vi "Run.vi"(7 "Team Index":i32, 8 "Column":i32, 9 "Row":i32, 10 "View":i32[](array[numeric]) caption="View (Team Index, -1: empty)", 11 "Uno In":refnum<class "Uno.lvclass">) -> (0 "Replicated":refnum<class "Square.lvclass">, 1 "Direction":T1, 2 "Action":T2, 3 "Square Out":refnum<class "Square.lvclass">)   [LabVIEW 2017, in "Uno.lvclass"]
uses:
  Uno.lvclass
  C:/Workspace/Endigit/SquareBattle/Square/Square.lvclass
  Square/Square.lvclass
  Type Defs/Action Enum.ctl
  Type Defs/Direction Enum.ctl
  Uno.lvclass/Uno.ctl
  Finish/Finish.lvclass
  SubVIs/Read-Only Globals.vi
  SubVIs/Read-Only Stats.vi
  SubVIs/Globals (private).vi
  Type Defs/SB Type Defs.lvlib
panel:
  # "NW\nN\nNE\nE\nSE\nS\nSW\nW"
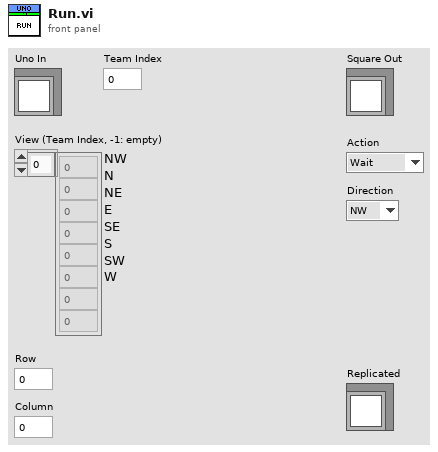
[diagram p1: front panel]
types:
  T1 = typedef "SB Type Defs.lvlib/Direction Enum.ctl" = enum16{"NW", "N", "NE", "E", "SE", "S", "SW", "W"}
  T2 = typedef "SB Type Defs.lvlib/Action Enum.ctl" = enum16{"Wait", "Move", "Attack", "Replicate"}
  T3 = typedef "Semaphore RefNum" = refnum<k1>
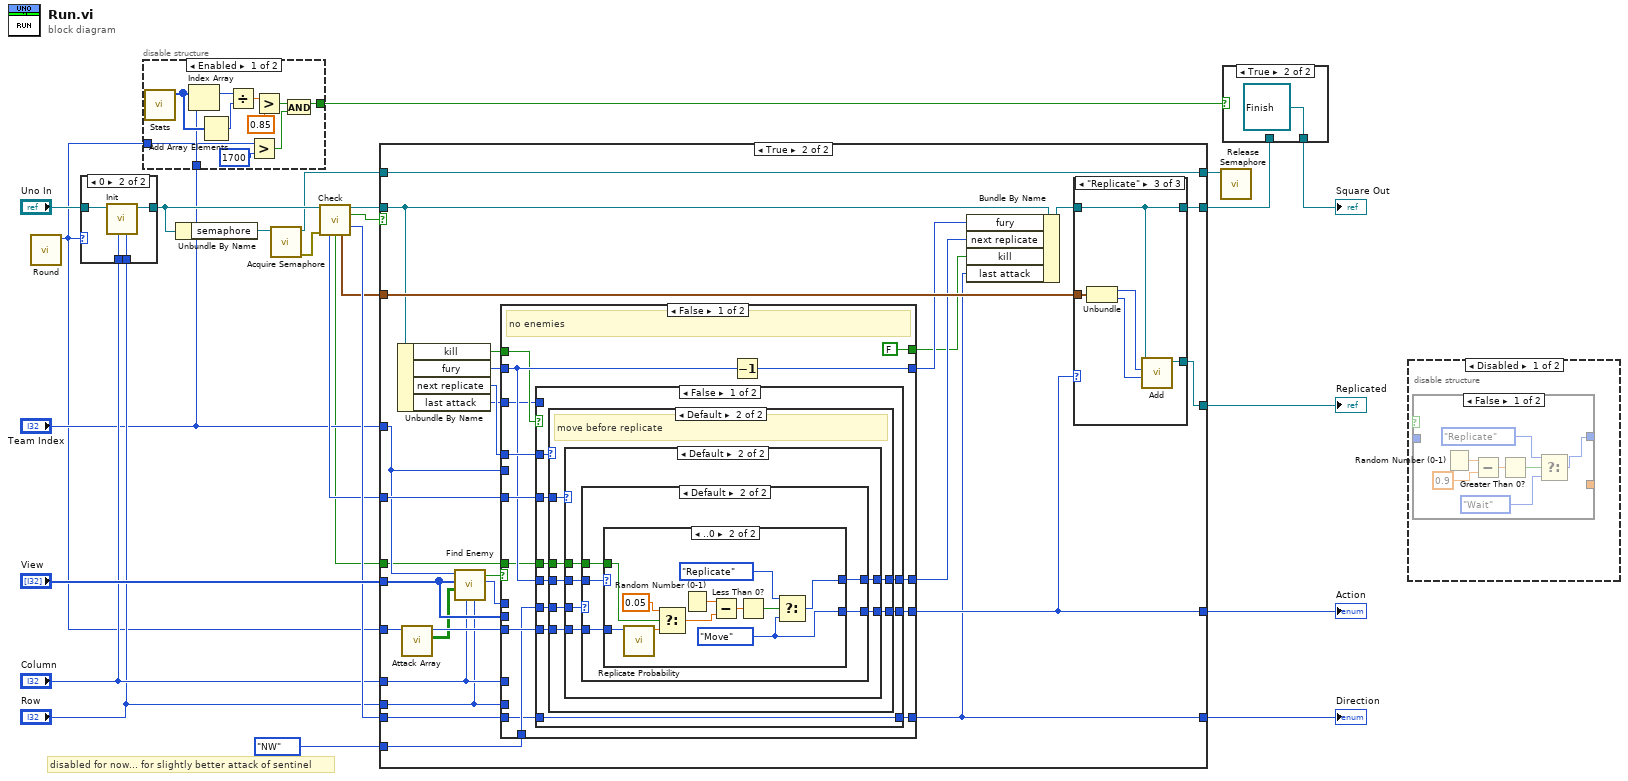
[diagram p0: block diagram]
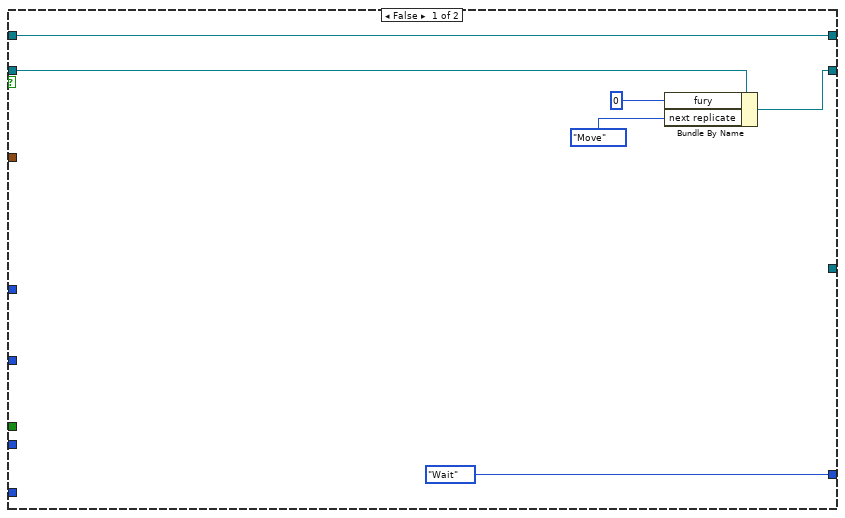
[diagram p4: hidden frame]
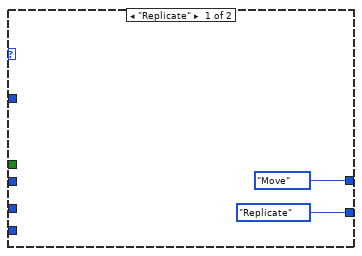
[diagram p5: hidden frame]
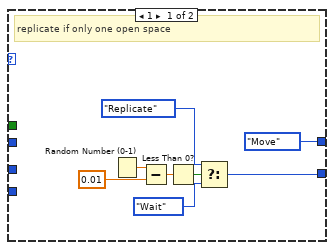
[diagram p6: hidden frame]
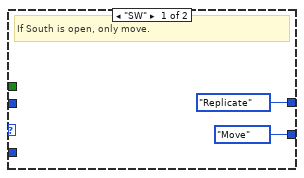
[diagram p7: hidden frame]
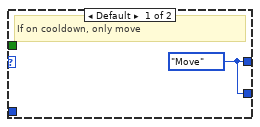
[diagram p8: hidden frame]
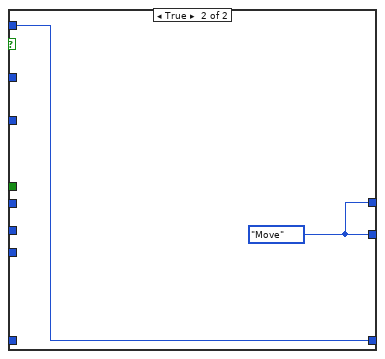
[diagram p9: hidden frame]
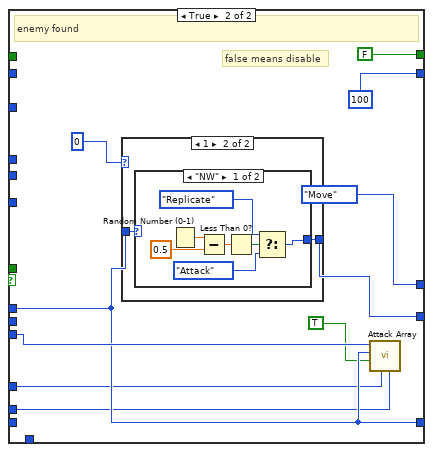
[diagram p10: hidden frame]
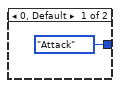
[diagram p11: hidden frame]
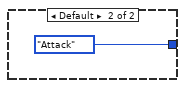
[diagram p12: hidden frame]
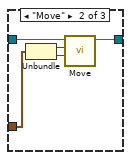
[diagram p14: hidden frame]
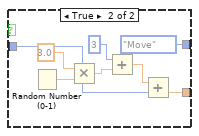
[diagram p15: hidden frame]
diagram:
  # "disabled for now... for slightly better attack of sentinel"
  n1 = call "Round.vi"() -> ("Round"=w2:i32)  [unwired: 11 in]
  n2 = case shown="0" w2 {
    tunnel: [w25 w29] -> w15
    tunnel: "Uno In" -> [w25 w28]
    tunnel: "Column" -> [_ w27]
    tunnel: "Row" -> [_ w26]
    frame Default {
    }
    frame 0 {
      n3 = call "Init.vi"("Y"=w26, "X"=w27, "Uno in"=w28) -> ("Uno out"=w29:refnum<class "Uno.lvclass">)  [unwired: 8 in]
    }
  }
  n4 = disable-structure shown="Enabled" {
    disable-tunnel: "Team Index" -> [w37 _]
    disable-tunnel: [w33 _] -> w5
    disable-tunnel: w2 -> [w31 _]
    frame Enabled {
      n5 = call "Stats.vi"() -> ("Squares"=w40:i32[])  [unwired: 7 in, 4 out]
      n6 = Index Array(array=w40, index=w37) -> (element=w38:i32)
      n7 = Add Array Elements(numeric array=w40) -> (sum=w39:i32)
      n8 = Divide(x=w38, y=w39) -> (x/y=w36:dbl)
      n9 = Greater?(x=w31, y=1700) -> (0:w32:bool)
      n10 = Greater?(x=w36, y=0.85) -> (0:w34:bool)
      n11 = And(x=w34, y=w32) -> (x .and. y?=w33:bool)
    }
    frame Disabled {
    }
  }
  n12 = Unbundle By Name(w15) -> ("semaphore"=w12:T3)
  n13 = call <vilib>:"Acquire Semaphore.vi"("semaphore"=w12) -> ("error out"=w10:errorcluster, "semaphore out"=w13:T3)  [unwired: 4 in, 1 out]
  n14 = call "Check.vi"("Uno in"=w15, "error in"=w10) -> ("Uno out"=w17:refnum<class "Uno.lvclass">, "run"=w20:bool, "open direction"=w19:T1, "open count"=w11:i16, "friendly zone"=w1:bool, "open coord"=w16:cluster{"X":i32, "Y":i32})  [unwired: 7 in, 1 out]
  n15 = case shown="True" w20 {
    tunnel: "Team Index" -> [_ w63]
    tunnel: [_ w51] -> w24
    tunnel: [Action_Enum."Wait" ("Action") w66] -> w23
    tunnel: "View" -> [_ w72]
    tunnel: w19 -> [_ w71]
    tunnel: [_ w62] -> w18
    tunnel: [w43 w70] -> w3
    tunnel: w17 -> [w44 w60]
    tunnel: w16 -> [_ w69]
    tunnel: [w45 w68] -> w14
    tunnel: w13 -> [w45 w68]
    tunnel: w11 -> [_ w64]
    tunnel: "Column" -> [_ w55]
    tunnel: "Row" -> [_ w54]
    tunnel: w2 -> [_ w57]
    tunnel: Direction_Enum."NW" ("Direction") -> [_ w52]
    tunnel: w1 -> [_ w47]
    frame False {
      n16 = Bundle By Name(cluster=w44, "fury"=0 ("fury cooldown"), "next replicate"=Action_Enum."Move") -> (w43:refnum<class "Uno.lvclass">)
    }
    frame True {
      n17 = Unbundle By Name(w60) -> ("kill"=w49:bool, "fury"=w59:i32, "next replicate"=w53:T2, "last attack"=w48:T1)
      n18 = call "Attack Array.vi"("Round"=w57) -> ("attack array"=w56:bool[][], "Round out"=w58:i32)  [unwired: 8 in, 1 out]
      n19 = call "Find Enemy.vi"("Y"=w54, "X"=w55, "attack array"=w56, "View"=w72, "Team Index"=w63) -> ("Direction"=w73:T1, "Found Enemy?"=w74:bool)  [unwired: 5 in]
      n20 = case shown="False" w74 {
        tunnel: [w79 w147] -> w51
        tunnel: w73 -> [_ w147]
        tunnel: [w88 w151] -> w66
        tunnel: w72 -> [_ _]
        tunnel: w71 -> [w78 _]
        tunnel: w58 -> [w87 w148]
        tunnel: [w86 Action_Enum."Move" ("f")] -> w65
        tunnel: w64 -> [w85 _]
        tunnel: w63 -> [_ _]
        tunnel: w53 -> [w84 _]
        tunnel: w55 -> [_ w145]
        tunnel: w54 -> [_ w144]
        tunnel: [w83 100 ("Team Index")] -> w61
        tunnel: w59 -> [w82 _]
        tunnel: w52 -> [w81 _]
        tunnel: [FALSE FALSE] -> w50
        tunnel: w49 -> [w77 _]
        tunnel: w48 -> [w76 _]
        tunnel: w47 -> [w75 _]
        frame False {
          # "no enemies"
          n21 = case shown="False" w77 {
            tunnel: [w97 w140] -> w88
            tunnel: w87 -> [w96 _]
            tunnel: [w95 w140] -> w86
            tunnel: w85 -> [w94 _]
            tunnel: w84 -> [w93 _]
            tunnel: w82 -> [w92 _]
            tunnel: w81 -> [w91 _]
            tunnel: [w90 w141] -> w79
            tunnel: w78 -> [w90 _]
            tunnel: w76 -> [_ w141]
            tunnel: w75 -> [w89 _]
            frame False {
              n22 = case shown="Default" w93 {
                tunnel: [Action_Enum."Replicate" ("f") w106] -> w97
                tunnel: w96 -> [_ w105]
                tunnel: w91 -> [_ w104]
                tunnel: [Action_Enum."Move" ("f") w103] -> w95
                tunnel: w94 -> [_ w102]
                tunnel: w92 -> [_ w101]
                tunnel: w89 -> [_ w100]
                frame "Replicate" {
                }
                frame Default {
                  # "move before replicate"
                  n23 = case shown="Default" w102 {
                    tunnel: [w107 w120] -> w106
                    tunnel: w105 -> [_ w119]
                    tunnel: w104 -> [_ w118]
                    tunnel: [Action_Enum."Move" ("f") w117] -> w103
                    tunnel: w101 -> [_ w116]
                    tunnel: w100 -> [_ w115]
                    frame 1 {
                      # "replicate if only one open space"
                      n24 = Random Number (0-1)() -> (number: 0 to 1=w112:dbl)
                      n25 = Subtract(x=w112, y=0.01) -> (x-y=w113:dbl)
                      n26 = Less Than 0?(x=w113) -> (x < 0?=w111:bool)
                      n27 = Select(t=Action_Enum."Replicate" ("Action"), s=w111, f=Action_Enum."Wait") -> (s? t:f=w107:T2)
                    }
                    frame Default {
                      n28 = case shown="Default" w118 {
                        tunnel: [Action_Enum."Move" ("f") w127] -> w120
                        tunnel: w119 -> [_ w125]
                        tunnel: [Action_Enum."Replicate" ("f") w126] -> w117
                        tunnel: w116 -> [_ w124]
                        tunnel: w115 -> [_ w123]
                        frame "SW" {
                          # "If South is open, only move."
                        }
                        frame Default {
                          n29 = case shown="..0" w124 {
                            tunnel: [w128 w135] -> w127
                            tunnel: [w128 w134] -> w126
                            tunnel: w125 -> [_ w133]
                            tunnel: w123 -> [_ w130]
                            frame Default {
                              w128 = Action_Enum."Move" ("f")
                              # "If on cooldown, only move"
                            }
                            frame ..0 {
                              w135 = Action_Enum."Move" ("f")
                              n30 = call "Replicate Probability.vi"("Round in"=w133) -> ("t"=w132:dbl)  [unwired: 10 in]
                              n31 = Select(t=0.05, s=w130, f=w132) -> (s? t:f=w131:dbl)
                              n32 = Random Number (0-1)() -> (number: 0 to 1=w138:dbl)
                              n33 = Subtract(x=w138, y=w131) -> (x-y=w139:dbl)
                              n34 = Less Than 0?(x=w139) -> (x < 0?=w137:bool)
                              n35 = Select(t=Action_Enum."Replicate" ("Action"), s=w137, f=w135) -> (s? t:f=w134:T2)
                            }
                          }
                        }
                      }
                    }
                  }
                }
              }
            }
            frame True {
              w140 = Action_Enum."Move" ("f")
            }
          }
          n36 = Decrement(x=w82) -> (x-1=w83:i32)
        }
        frame True {
          # "false means disable"
          # "enemy found"
          n37 = case shown="1" 0 ("Team Index") {
            tunnel: [Action_Enum."Attack" ("Action") w154] -> w151
            tunnel: w147 -> [_ w153]
            frame 0, Default {
            }
            frame 1 {
              n38 = case shown="\"NW\"" w153 {
                tunnel: [w156 Action_Enum."Attack" ("Action")] -> w154
                frame "NW" {
                  n39 = Random Number (0-1)() -> (number: 0 to 1=w160:dbl)
                  n40 = Subtract(x=w160, y=0.5) -> (x-y=w161:dbl)
                  n41 = Less Than 0?(x=w161) -> (x < 0?=w159:bool)
                  n42 = Select(t=Action_Enum."Replicate" ("Action"), s=w159, f=Action_Enum."Attack") -> (s? t:f=w156:T2)
                }
                frame Default {
                }
              }
            }
          }
          n43 = call "Attack Array.vi"("Y"=w144, "X"=w145, "add attack"=TRUE, "Direction"=w147, "Round"=w148) -> ()  [unwired: 4 in, 3 out]
        }
      }
      n44 = Bundle By Name(cluster=w60, "fury"=w61, "next replicate"=w65, "kill"=w50, "last attack"=w51) -> (w67:refnum<class "Uno.lvclass">)
      n45 = case shown="\"Replicate\"" w66 {
        tunnel: [_ _ w173] -> w62
        tunnel: [w163 w167 w169] -> w70
        tunnel: w67 -> [w163 w168 w169]
        tunnel: w69 -> [_ w166 w172]
        frame Default {
        }
        frame "Move" {
          n46 = Unbundle(w166) -> ("X"=w165:i32, "Y"=w164:i32)
          n47 = call "Move.vi"("Y"=w164, "X"=w165, "Uno in"=w168) -> ("Uno out"=w167:refnum<class "Uno.lvclass">)  [unwired: 7 in, 1 out]
        }
        frame "Replicate" {
          n48 = Unbundle(w172) -> ("X"=w171:i32, "Y"=w170:i32)
          n49 = call "Add.vi"("Y"=w170, "X"=w171, "Uno in"=w169) -> ("Uno out"=w173:refnum<class "Uno.lvclass">)  [unwired: 7 in, 1 out]
        }
      }
    }
  }
  "Action" <- w23
  "Direction" <- w24
  "Replicated" <- w18
  n50 = call <vilib>:"Release Semaphore.vi"("semaphore"=w14) -> ()  [unwired: 5 in, 2 out]
  n51 = case shown="True" w5 {
    tunnel: [w174 refnum<class "Finish.lvclass"> refnum ("Finish.lvclass")] -> w4
    tunnel: w3 -> [w174 _]
    frame False {
    }
    frame True {
    }
  }
  "Square Out" <- w4
  n52 = disable-structure shown="Disabled" {
    frame Disabled {
      n53 = case shown="False" {
        selector: _ -> [_ _]
        tunnel: _ -> [_ w189]
        tunnel: [_ w188] -> _
        tunnel: [w177 Action_Enum."Move" ("Action")] -> _
        frame False {
          n54 = Random Number (0-1)() -> (number: 0 to 1=w182:dbl)
          n55 = Subtract(x=w182, y=0.9) -> (x-y=w180:dbl)
          n56 = Greater Than 0?(x=w180) -> (x > 0?=w179:bool)
          n57 = Select(t=Action_Enum."Replicate" ("Action"), s=w179, f=Action_Enum."Wait") -> (s? t:f=w177:T2)
        }
        frame True {
          n58 = Random Number (0-1)() -> (number: 0 to 1=w186:dbl)
          n59 = Multiply(x=3.0, y=w186) -> (x*y=w184:dbl)
          n60 = Add(x=3 ("Team Index"), y=w184) -> (x+y=w183:dbl)
          n61 = Add(x=w183, y=w189) -> (x+y=w188:dbl)
        }
      }
    }
    frame Enabled {
    }
  }
